vi "写入Events.vi"(8 "error in (no error)":errorcluster caption="错误输入（无错误）", 10 "Events":cluster{"Stop":refnum<user-event>}, 11 "2601B输入":refnum<class "2601B.lvclass">) -> (0 "error out":errorcluster caption="错误输出", 3 "2601B输出":refnum<class "2601B.lvclass">)   [LabVIEW 2020, in "2601B.lvclass"]
uses:
  2601B.lvclass
  2601B.lvclass/2601B.ctl
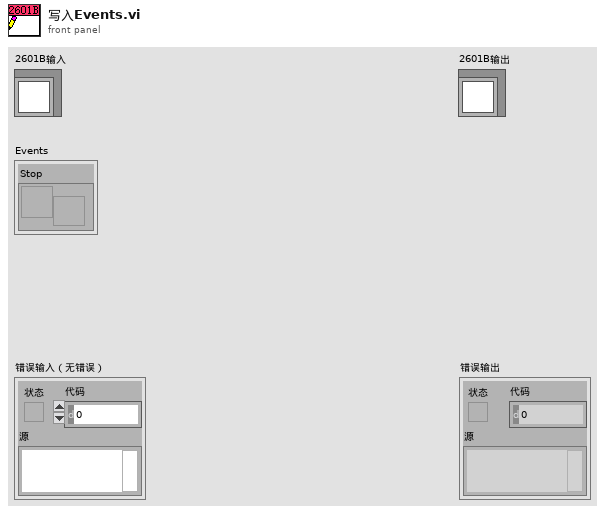
[diagram p1: front panel]
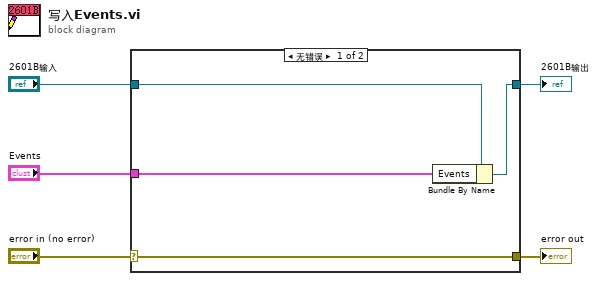
[diagram p0: block diagram]
diagram:
  n1 = case shown="无错误" "error in (no error)" {
    selector: "error in (no error)" -> [w9 w10]
    tunnel: [w9 w10] -> w4
    tunnel: [w7 w11] -> w2
    tunnel: "2601B输入" -> [w8 w11]
    tunnel: "Events" -> [w6 _]
    frame No Error {
      n2 = Bundle By Name(cluster=w8, "Events"=w6) -> (w7:refnum<class "2601B.lvclass">)
    }
    frame Error {
    }
  }
  "error out" <- w4
  "2601B输出" <- w2
